vi "Bounce Window_Modify User.vi"(11 "User Account Data In":T1={"帳號 :"="", "權限等級："=enum."開發人員", "建立時間："="", "修改時間："="", "到期時間："="", "狀態："=enum."可使用", "期限："=enum."一天", "密碼："=""}) -> (2 "是否新增":bool, 3 "User Account Data":T1={"帳號 :"="", "權限等級："=enum."開發人員", "建立時間："="", "修改時間："="", "到期時間："="", "狀態："=enum."可使用", "期限："=enum."一天", "密碼："=""})   [LabVIEW 2015]
uses:
  <vilib>/Utility/miscctls.llb/LVPointTypeDef.ctl
panel:
  out "到期日期：":string
  in  "取消":bool
  in  "狀態：":T3
  in  "增加天數：":T4
  in  "確認":bool
  in  "權限等級：":T2
  out "帳號：":string
  # "修改帳號"
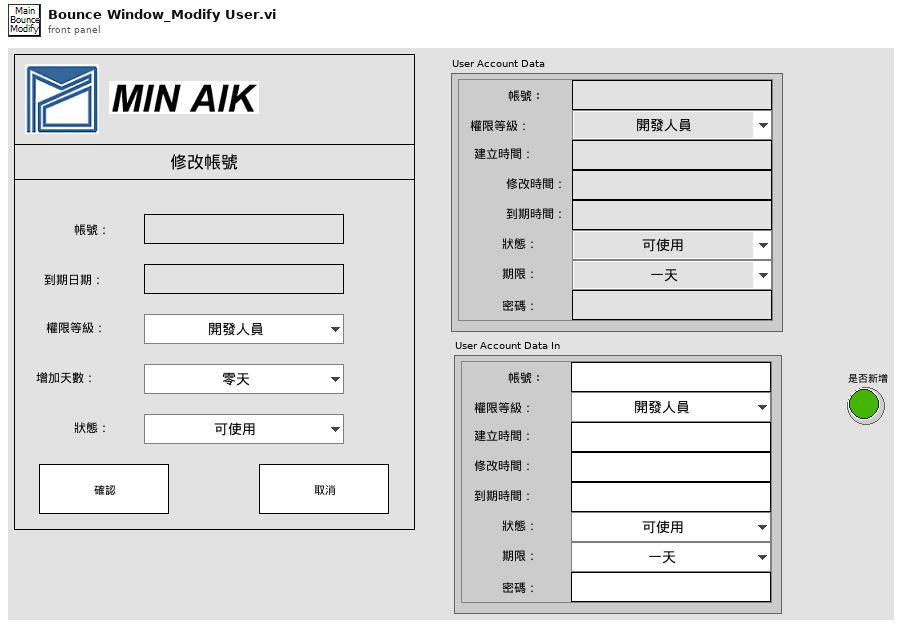
[diagram p1: front panel]
types:
  T1 = typedef "Control_User account_Data.ctl" = cluster{"帳號 :":string, "權限等級：":T2, "建立時間：":string, "修改時間：":string, "到期時間：":string, "狀態：":T3, "期限：":T4, "密碼：":string}
  T2 = typedef "Control_User account_Permissions.ctl" = enum16{"開發人員", "管理者", "工程師", "作業員"}
  T3 = typedef "Control_User Accounts_Status.ctl" = enum16{"可使用", "不可使用"}
  T4 = typedef "Control_User account_Date.ctl" = enum16{"零天", "一天", "七天", "一個月", "一年", "三年"}
  T5 = typedef "LVPointTypeDef.ctl" = cluster{"Horizontal":i16, "Vertical":i16}
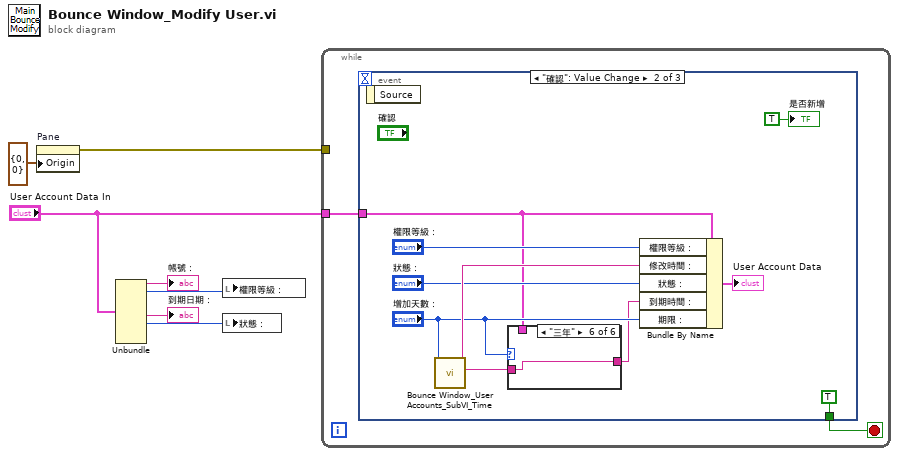
[diagram p0: block diagram]
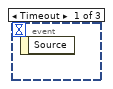
[diagram p2: hidden frame]
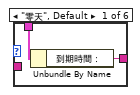
[diagram p3: hidden frame]
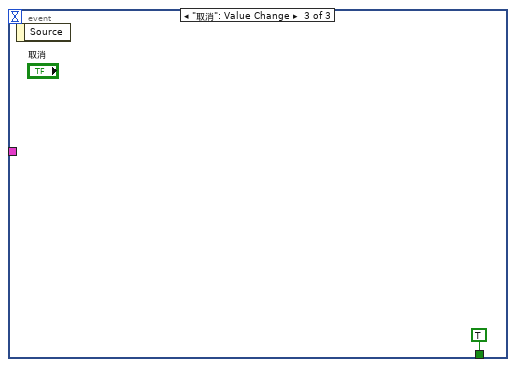
[diagram p8: hidden frame]
diagram:
  n1 = property on="Pane" class="Pane"("Origin"=T5 {"Horizontal"=0, "Vertical"=0}) -> (error out=w7:errorcluster)  [unwired: 2 in, 1 out]
  n2 = Unbundle("User Account Data In") -> ("帳號 :"=→"帳號：":string, "權限等級："=w4:T2, "到期時間："=→"到期日期：":string, "狀態："=w5:T3)  [unwired: 4 out]
  n3 = local write "權限等級："(w4) -> ()
  n4 = local write "狀態："(w5) -> ()
  n5 = while {
    tunnel: "User Account Data In" -> [w8]
    tunnel: w7 -> [_]
    stop <- w9 stop-if-true
    n6 = event shown="[1] \"確認\": Value Change" {
      selector: _ -> [_ _ _]
      dyn-events: _ -> [_ _ _]
      timeout: _ -> [_ _ _]
      tunnel: [_ TRUE TRUE] -> w9
      tunnel: w8 -> [_ w11 _]
      event Timeout {
        n7 = event-data() -> ()  [unwired: 1 in, 1 out]
      }
      event "確認": Value Change {
        n8 = event-data() -> ()  [unwired: 1 in, 1 out]
        n9 = call "Bounce Window_User Accounts_SubVI_Time.vi"("期限："="增加天數：") -> ("期限"=w12:string, "目前時間"=w18:string)  [unwired: 9 in]
        n10 = case shown="\"三年\"" "增加天數：" {
          tunnel: w12 -> [_ w22 w23 w24 w25 w26]
          tunnel: w11 -> [w21 _ _ _ _ _]
          tunnel: [w20 w22 w23 w24 w25 w26] -> w10
          frame "零天", Default {
            n11 = Unbundle By Name(w21) -> ("到期時間："=w20:string)
          }
          frame "一天" {
          }
          frame "七天" {
          }
          frame "一個月" {
          }
          frame "一年" {
          }
          frame "三年" {
          }
        }
        n12 = Bundle By Name(cluster=w11, "權限等級："="權限等級：", "修改時間："=w18, "狀態："="狀態：", "到期時間："=w10, "期限："="增加天數：") -> (→"User Account Data":T1)
        "是否新增" <- TRUE ("是否新增")
      }
      event "取消": Value Change {
        n13 = event-data() -> ()  [unwired: 1 in, 1 out]
      }
    }
  }
